vi "_UpdateDAQFIFOOnlineDisplay_HH.vi"(0 "Show Decay":refnum<vi>, 1 "Show MCS":refnum<vi>, 2 "Counts":refnum<vi>, 3 "Decay":refnum<vi>, 4 "MCS":refnum<vi>, 5 "rawdata":u32[](array[numeric]), 6 "count (read)":u32, 7 "operation":enum16{"initilalize", "update"}(ring)) -> ()   [LabVIEW 2009]
panel:
  in  "Show Decay Substitute":bool
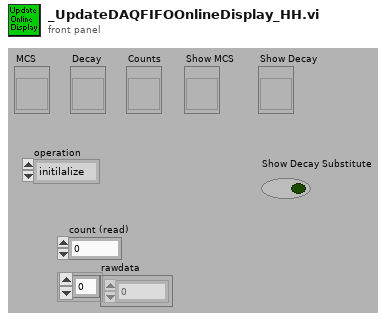
[diagram p1: front panel]
types:
  T1 = cluster{"Binning [µs]":dbl, "Overflow Constant":dbl, "Macrotime Cycle":dbl, "Binning Cycle":dbl, "Current Decay":i32, "Bins Used":u32, "Decay Used":i32, "Total Count":u32, "Gap Count":u32, "Invalid Count":u32}
  T2 = typedef "FIFOSettings.ctt" = cluster{"Measurement":cluster{"Binning (ms)":sgl, "External Trigger Condition":u16, "Stop Condition:":u16, "Stop Count":dbl, "Buffer Size (Photons)":u32, "No of Channels":u16, "Ext Latch Delay":i16}, "ADC":cluster{"Binning (HH)":i16, "Dither Range":i16, "Count Increment":i16, "Mode":u16}, "SYNC":cluster{"SYNC ZC Level (mV)":sgl, "SYNC Freq Divider":u16, "SYNC Holdoff (ps)":sgl, "SYNC Threshold (mV)":sgl}, "TAC":cluster{"TAC Range (ns)":sgl, "TAC Gain":i16, "TAC Offset (%)":sgl, "TAC Limit Low (%)":sgl, "TAC Limit High (%)":sgl}, "Ch 2":cluster{"Ch2 ZC Level (mV)":sgl, "Ch2 Holdoff (ps)":sgl, "Ch2 Threshold (mV)":sgl}, "Ch 3":cluster{"Ch3 ZC Level (mV)":sgl, "Ch3 Holdoff (ps)":sgl, "Ch3 Threshold (mV)":sgl}, "Ch 4":cluster{"Ch4 ZC Level (mV)":sgl, "Ch4 Holdoff (ps)":sgl, "Ch4 Threshold (mV)":sgl}, "Ch1":cluster{"Ch1 ZC Level (mV)":sgl, "Ch1 Holdoff (ps)":sgl, "Ch1 Threshold (mV)":sgl}}
  T3 = cluster{"Total Count":u32, "Gap Count":u32, "Invalid Count":u32}
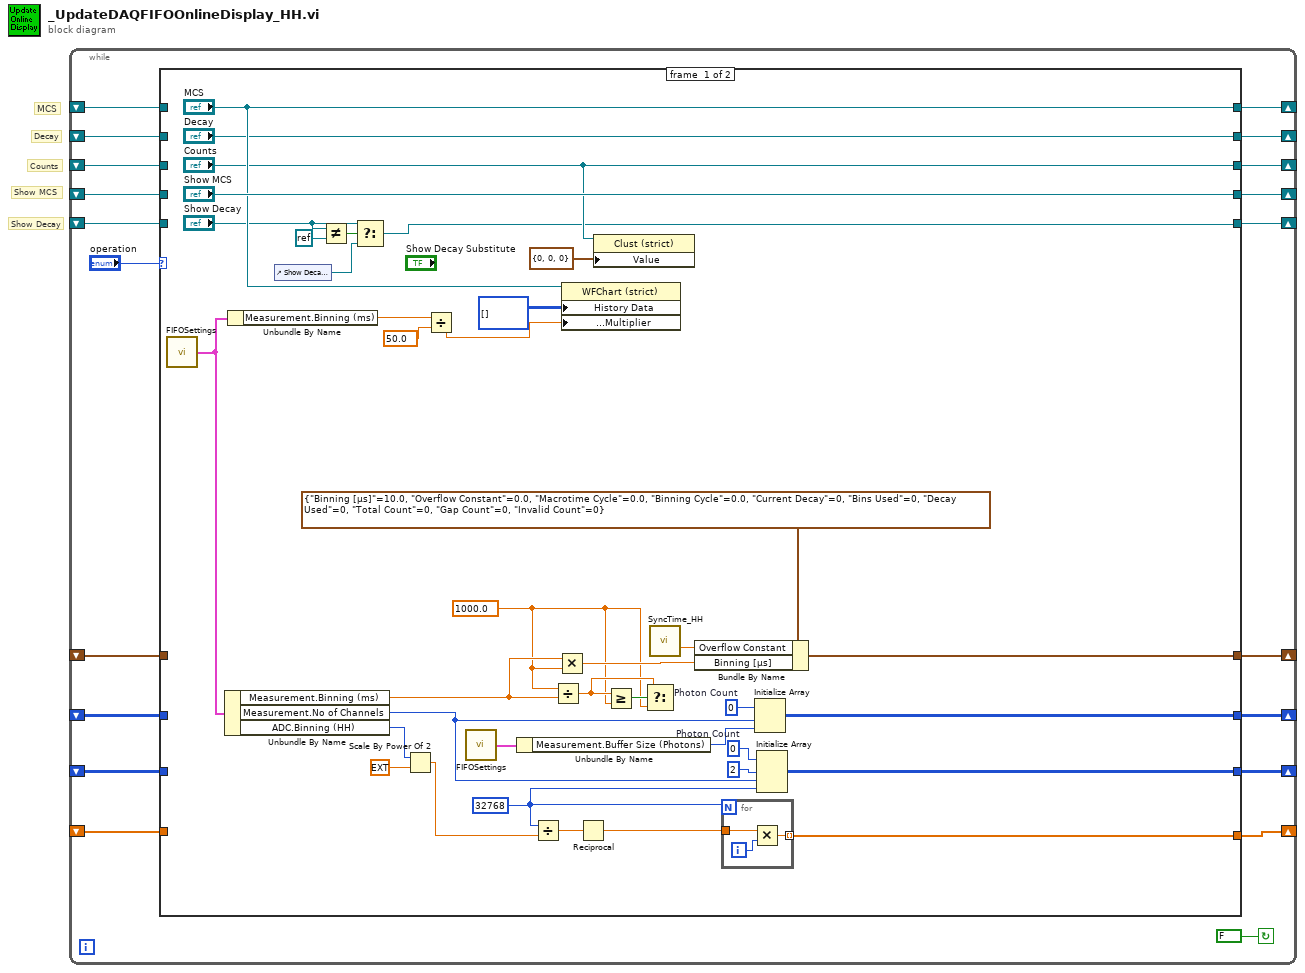
[diagram p0: block diagram]
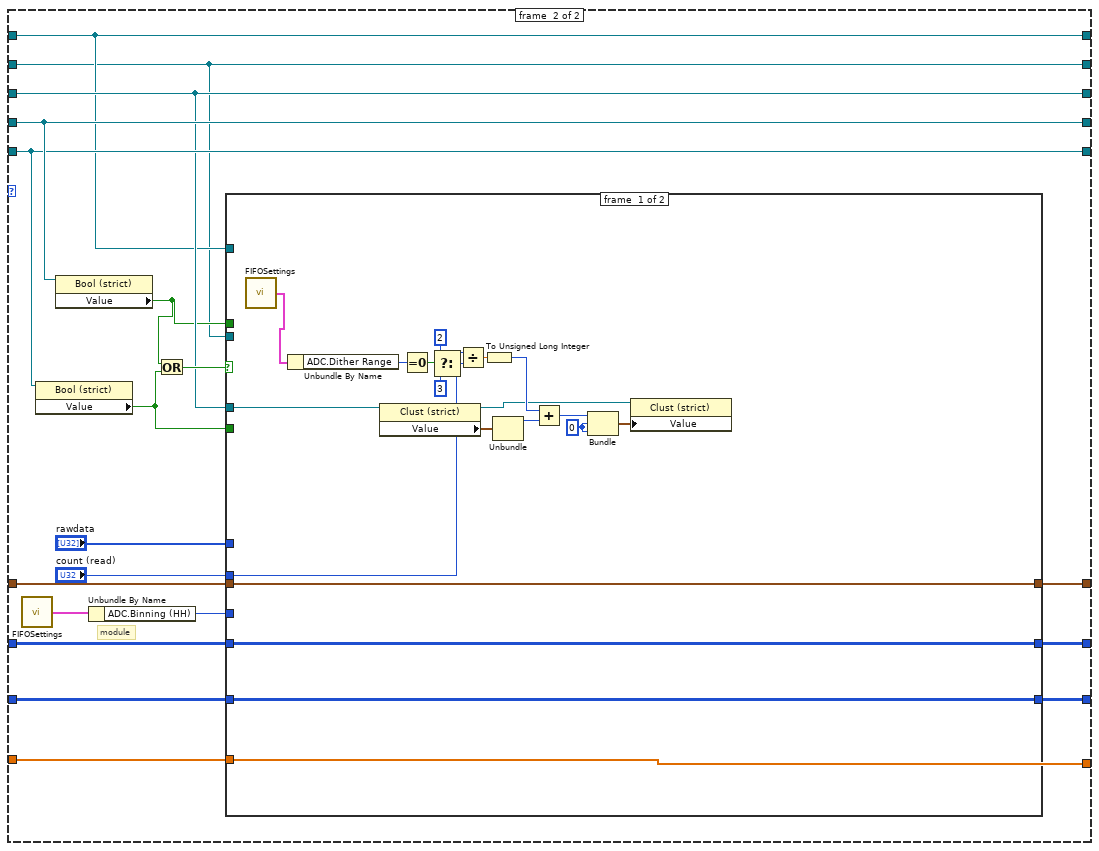
[diagram p2: hidden frame]
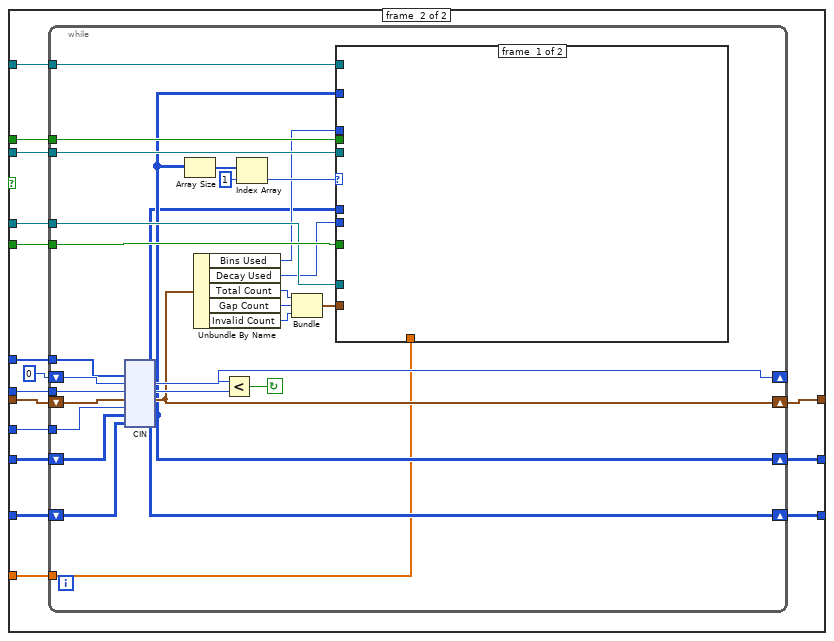
[diagram p3: hidden frame]
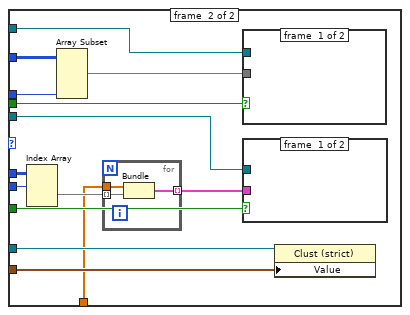
[diagram p4: hidden frame]
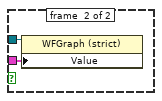
[diagram p5: hidden frame]
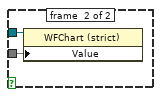
[diagram p6: hidden frame]
diagram:
  # "Show Decay"
  # "Show MCS"
  # "Counts"
  # "Decay"
  # "MCS"
  n1 = while {
    shift-right: [w19] -> _
    shift-left: _ -> [w14]
    shift-right: [w18] -> _
    shift-left: _ -> [w13]
    shift-right: [w17] -> _
    shift-left: _ -> [w12]
    shift-right: [w16] -> _
    shift-left: _ -> [w11]
    shift-right: [w15] -> _
    shift-left: _ -> [w10]
    shift-right: [w8] -> _
    shift-left: _ -> [w4]
    shift-right: [w7] -> _
    shift-left: _ -> [w3]
    shift-right: [w6] -> _
    shift-left: _ -> [w2]
    shift-right: [w5] -> _
    shift-left: _ -> [w1]
    stop <- FALSE continue-if-true
    n2 = case shown="\"initilalize\", Default" "operation" {
      tunnel: ["MCS" w72] -> w19
      tunnel: ["Decay" w71] -> w18
      tunnel: ["Counts" w77] -> w17
      tunnel: ["Show MCS" w80] -> w16
      tunnel: [w45 w79] -> w15
      tunnel: w14 -> [_ w72]
      tunnel: w13 -> [_ w71]
      tunnel: w12 -> [_ w77]
      tunnel: w11 -> [_ w80]
      tunnel: w10 -> [_ w79]
      tunnel: [w36 w70] -> w8
      tunnel: [w35 w69] -> w7
      tunnel: [w34 w68] -> w6
      tunnel: [w33 w64] -> w5
      tunnel: w4 -> [_ w67]
      tunnel: w3 -> [_ w66]
      tunnel: w2 -> [_ w65]
      tunnel: w1 -> [_ w64]
      frame #0 {
        w31 = 1000.0 ("y")
        w27 = u32 32768
        w43 = u32 0  # Photon Count
        w44 = u32 0  # Photon Count
        n3 = call "FIFOSettings.vi"() -> ("FIFO Settings(out)"=w30:T2)  [unwired: 2 in]
        n4 = Unbundle By Name(w30) -> ("Measurement.Binning (ms)"=w41:sgl, "Measurement.No of Channels"=w39:u16, "ADC.Binning (HH)"=w25:i16)
        n5 = Unbundle By Name(w30) -> ("Measurement.Binning (ms)"=w55:sgl)
        n6 = control-ref of="Show Decay Substitute"() -> (w46:refnum<vi>)
        n7 = Not Equal?(x="Show Decay", y=refnum<k0> refnum) -> (x != y?=w48:bool)
        n8 = Select(t="Show Decay", s=w48, f=w46) -> (s? t:f=w45:refnum<vi>)
        n9 = Scale By Power Of 2(n=w25, x=ext 1.0) -> (x*2^n=w24:ext)
        n10 = Divide(x=w55, y=sgl 50.0) -> (x/y=w54:sgl)
        n11 = call "FIFOSettings.vi"() -> ("FIFO Settings(out)"=w22:T2)  [unwired: 2 in]
        n12 = Unbundle By Name(w22) -> ("Measurement.Buffer Size (Photons)"=w21:u32)
        n13 = Divide(x=w27, y=w24) -> (x/y=w26:ext)
        n14 = Divide(x=w31, y=w41) -> (x/y=w32:dbl)
        n15 = Multiply(x=w41, y=w31) -> (x*y=w42:dbl)
        n16 = property class="WFChart (strict)"(reference="MCS", "History Data"=u32[][] [] ("MCS"), "X Scale.Offset and Multiplier:Multiplier"=w54) -> ()  [unwired: 1 in, 2 out]
        n17 = Reciprocal(x=w26) -> (1/x=w28:ext)
        n18 = property class="Clust (strict)"(reference="Counts", "Value"=cluster{"Total":u32, "Gap":u32, "Invalid":u32} {"Total"=0, "Gap"=0, "Invalid"=0} ("Counts")) -> ()  [unwired: 1 in, 2 out]
        n19 = Greater Or Equal?(x=w32, y=w31) -> (x >= y?=w38:bool)
        n20 = Select(t=w32, s=w38, f=w31) -> ()  [unwired: 1 out]
        n21 = call "SyncTime_HH.vi"() -> ("OverFlowConstant80Mhz(µs)"=w29:dbl)
        n22 = Bundle By Name(cluster=T1 {"Binning [µs]"=10.0, "Overflow Constant"=0.0, "Macrotime Cycle"=0.0, "Binning Cycle"=0.0, "Current Decay"=0, "Bins Used"=0, "Decay Used"=0, "Total Count"=0, "Gap Count"=0, "Invalid Count"=0}, "Overflow Constant"=w29, "Binning [µs]"=w42) -> (w36:T1)
        n23 = for {
          N: w27 -> [_]
          tunnel: [w60] -> w33 mode=indexing
          tunnel: w28 -> [w59]
          i -> [w61]
          n24 = Multiply(x=w59, y=w61) -> (x*y=w60:ext)
        }
        n25 = Initialize Array(w44, w39, w21) -> (w35:u32[][])
        n26 = Initialize Array(w43, u32 2 ("y"), w39, w27) -> (w34:u32[][][])
      }
      frame #1 {
        # "module"
        n27 = call "FIFOSettings.vi"() -> ("FIFO Settings(out)"=w62:T2)  [unwired: 2 in]
        n28 = property class="Bool (strict)"(reference=w79) -> ("Value"=w73:bool)  [unwired: 1 in, 2 out]
        n29 = property class="Bool (strict)"(reference=w80) -> ("Value"=w74:bool)  [unwired: 1 in, 2 out]
        n30 = Unbundle By Name(w62) -> ("ADC.Binning (HH)"=w63:i16)
        n31 = Or(x=w74, y=w73) -> (x .or. y?=w78:bool)
        n32 = case shown="True" w78 {
          tunnel: w77 -> [w87 w110]
          tunnel: "count (read)" -> [w85 w114]
          tunnel: "rawdata" -> [_ w113]
          tunnel: w74 -> [_ w112]
          tunnel: w73 -> [_ w111]
          tunnel: w72 -> [_ w109]
          tunnel: w71 -> [_ w108]
          tunnel: [w84 w107] -> w70
          tunnel: [w83 w106] -> w69
          tunnel: [w82 w105] -> w68
          tunnel: w67 -> [w84 w104]
          tunnel: w66 -> [w83 w103]
          tunnel: w65 -> [w82 w102]
          tunnel: w64 -> [_ w101]
          tunnel: w63 -> [_ w100]
          frame #0 {
            w96 = u32 0 ("element")
            n33 = call "FIFOSettings.vi"() -> ("FIFO Settings(out)"=w81:T2)  [unwired: 2 in]
            n34 = Unbundle By Name(w81) -> ("ADC.Dither Range"=w90:i16)
            n35 = property on="Property Node" class="Clust (strict)"(reference=w87) -> (reference out=w86:refnum<vi>, "Value"=w98:cluster{"Total":u32, "Gap":u32, "Invalid":u32})  [unwired: 1 in, 1 out]
            n36 = Equal To 0?(x=w90) -> (x = 0?=w91:bool)
            n37 = Select(t=2, s=w91, f=3) -> (s? t:f=w94:i32)
            n38 = Divide(x=w85, y=w94) -> (x/y=w95:dbl)
            n39 = To Unsigned Long Integer(number=w95) -> (unsigned 32bit integer=w89:u32)
            n40 = Unbundle(w98) -> ("Total"=w88:u32)  [unwired: 2 out]
            n41 = Add(x=w89, y=w88) -> (x+y=w97:u32)
            n42 = Bundle(w97, "element"=w96, "element"=w96) -> (w99:cluster{u32, "element":u32, "element":u32})  [unwired: 1 in]
            n43 = property on="Property Node" class="Clust (strict)"(reference=w86, "Value"=w99) -> ()  [unwired: 1 in, 2 out]
          }
          frame #1 {
            n44 = while {
              shift-right: [w131] -> _
              shift-left: u32 0 ("offset (output)") -> [w133]
              tunnel: w114 -> [w132]
              tunnel: w113 -> [w123]
              tunnel: w112 -> [w139]
              tunnel: w111 -> [w138]
              tunnel: w110 -> [w137]
              tunnel: w109 -> [w136]
              tunnel: w108 -> [w135]
              shift-right: [w124] -> w107
              shift-left: w104 -> [w130]
              shift-right: [w121] -> w106
              shift-left: w103 -> [w129]
              shift-right: [w119] -> w105
              shift-left: w102 -> [w128]
              tunnel: w101 -> [w118]
              tunnel: w100 -> [w116]
              stop <- w134 continue-if-true
              n45 = cin(w123, w133, w132, w130, w116, w129, w128) -> (w131:u32, w124:T1, w121:u32[][], w119:u32[][][])  [unwired: 3 in]
              n46 = Array Size(array=w121) -> (size(s)=w141:i32[])
              n47 = Unbundle By Name(w124) -> ("Bins Used"=w120:u32, "Decay Used"=w117:i32, "Total Count"=w127:u32, "Gap Count"=w126:u32, "Invalid Count"=w125:u32)
              n48 = Less?(x=w131, y=w132) -> (x < y?=w134:bool)
              n49 = Index Array(array=w141, index=1) -> (element=w140:i32)
              n50 = Bundle("Total Count"=w127, "Gap Count"=w126, "Invalid Count"=w125) -> (w122:T3)  [unwired: 1 in]
              n51 = case shown="1, Default" w140 {
                tunnel: w139 -> [_ w156]
                tunnel: w138 -> [_ w155]
                tunnel: w137 -> [_ w154]
                tunnel: w122 -> [_ w153]
                tunnel: w136 -> [_ w152]
                tunnel: w135 -> [_ w151]
                tunnel: w121 -> [_ w150]
                tunnel: w120 -> [_ w148]
                tunnel: w119 -> [_ w147]
                tunnel: w118 -> [_ w145]
                tunnel: w117 -> [_ w143]
                frame #0 {
                }
                frame #1 {
                  n52 = Index Array(array=w147, index (dim 0)=w143) -> (element=w146:u32[][])  [unwired: 2 in]
                  n53 = Array Subset(array=w150, length (col)=w148) -> (w149:u32[][])  [unwired: 3 in]
                  n54 = for {
                    tunnel: w145 -> [w159]
                    tunnel: [w158] -> w144 mode=indexing
                    tunnel: w146 -> [w157] mode=indexing
                    n55 = Bundle(w159, w157) -> (w158:cluster{ext[], u32[]})  [unwired: 1 in]
                  }
                  n56 = case shown="True" w156 {
                    tunnel: w152 -> [_ w163]
                    tunnel: w149 -> [_ w162]
                    frame #0 {
                    }
                    frame #1 {
                      n57 = property on="Property Node" class="WFChart (strict)"(reference=w163, "Value"=w162) -> ()  [unwired: 1 in, 2 out]
                    }
                  }
                  n58 = case shown="True" w155 {
                    tunnel: w151 -> [_ w161]
                    tunnel: w144 -> [_ w160]
                    frame #0 {
                    }
                    frame #1 {
                      n59 = property on="Property Node" class="WFGraph (strict)"(reference=w161, "Value"=w160) -> ()  [unwired: 1 in, 2 out]
                    }
                  }
                  n60 = property on="Property Node" class="Clust (strict)"(reference=w154, "Value"=w153) -> ()  [unwired: 1 in, 2 out]
                }
              }
            }
          }
        }
      }
    }
  }
